vi "JSON Config Time Vector.vi"(7 "Expected Class":refnum<class "Abs_Time.lvclass">, 8 "error in (no error)":errorcluster, 11 "Test Value":timestamp) -> (0 "error out":errorcluster)   [LabVIEW 2021]
uses:
  Source/Abs_Types/Time/Abs_Time.lvclass
  C:/New folder/LV_Abstract/LV_Abstract/Source/Abs_Types/Type/Abs_Type.lvclass
  Source/Abs_Types/Time/Simple Read.vi
  Source/Constants/Support/Time/Time.vi
  <vilib>/addons/_JKI Toolkits/Caraya/classes/Assert/Assert Less_Variant.vi
  <vilib>/addons/_JKI Toolkits/Caraya/classes/Assert/Assert Equal Type_Variant.vi
  Source/Constants/Support/Time/Const_Time.lvclass
  <vilib>/addons/_JKI Toolkits/Caraya/classes/Assert/Assert.lvclass
  <vilib>/addons/_JKI Toolkits/Caraya/classes/Test/Test.lvclass
  <vilib>/Utility/Data Type/NI_Data Type.lvlib
  Source/Abs_Types/Type/Abs_Type.lvclass
panel:
  out "JSON":string
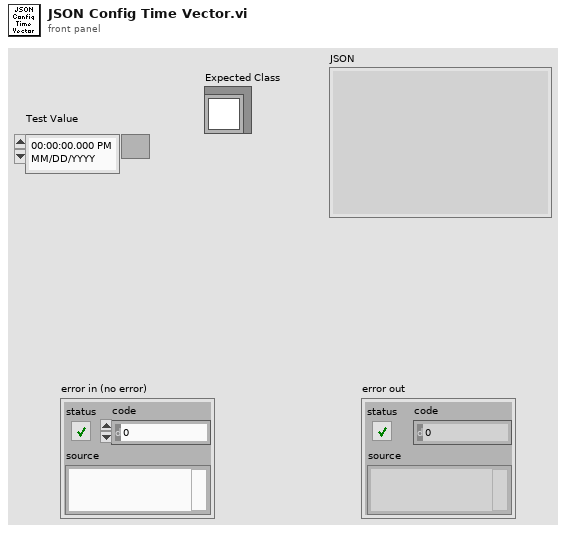
[diagram p1: front panel]
types:
  T1 = typedef "NI_Data Type.lvlib/Data Type.ctl" = enum8{"Invalid Type", "Void", "I8", "I16", "I32", "I64", "U8", "U16", "U32", "U64", "Single Float", "Double Float", "Extended Float", "Single Complex", "Double Complex", "Extended Complex", "Enum U8", "Enum U16", "Enum U32", "Enum U64", "Single Float With Unit", "Double Float With Unit", "Extended Float With Unit", "Single Complex with Unit", "Double Complex with Unit", "Extended Complex with Unit", "Boolean", "String", "Path", "Picture", "Tag", "Array", "Cluster", "Variant", "LV Variant", "Waveform", "Timestamp", "Digital Waveform", "Digital Data", "ExpressData", "Refnum", "External Data", "VI", "Poly VI", "LabVIEW Class Instance", "Fixed Point", "Set Collection", "Map Collection"}
  T2 = typedef "Abs_Time.lvclass/Type.ctl" = timestamp
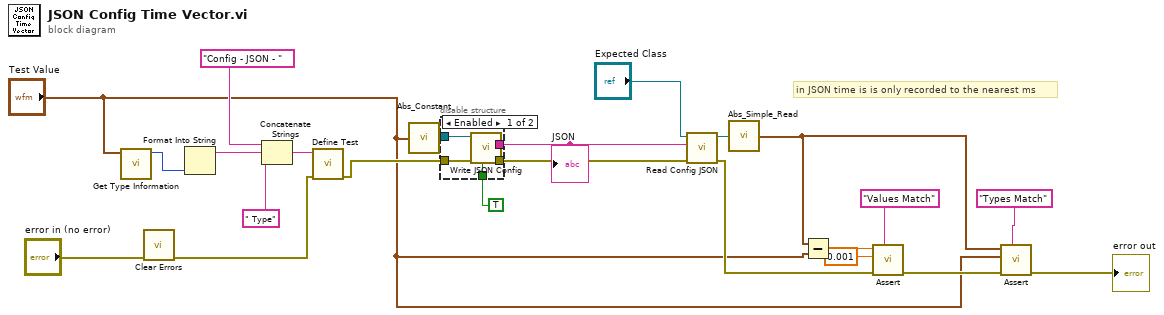
[diagram p0: block diagram]
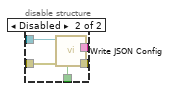
[diagram p2: hidden frame]
diagram:
  # "in JSON time is is only recorded to the nearest ms"
  n1 = call <vilib>:"Get Type Information.vi"("variant"="Test Value") -> ("type"=w14:T1)  [unwired: 6 in, 4 out]
  n2 = call <vilib>:"Clear Errors.vi"("error in (no error)"="error in (no error)") -> ("error out"=w9:errorcluster)  [unwired: 5 in, 1 out]
  n3 = Format Into String(w14) -> (resulting string=w13:string)  [unwired: 3 in, 1 out]
  n4 = Concatenate Strings("Config - JSON - " ("string"), w13, " Type" ("string")) -> (w12:string)
  n5 = call <vilib>:"Define Test.vi"("error in (no error)"=w9, "Label (VI Title)"=w12) -> ("error out"=w15:errorcluster)  [unwired: 8 in, 1 out]
  n6 = call-poly "Abs_Constant.vi"("Value"="Test Value") -> ("Constant"=w23:refnum<class "Const_Time.lvclass">)  [unwired: 4 in]
  n7 = disable-structure shown="Enabled" {
    disable-tunnel: w23 -> [w28 w33]
    disable-tunnel: TRUE ("Include Class Name") -> [w27 w32]
    disable-tunnel: [w26 w31] -> w21
    disable-tunnel: [w25 w30] -> w20
    disable-tunnel: w15 -> [w24 w29]
    frame Enabled {
      n8 = call-dynamic "Write JSON Config.vi"("Pretty Print?"=w27, "error in (no error)"=w24, "Const_Time in"=w28) -> ("error out"=w25:errorcluster, "JSON"=w26:string)  [unwired: 6 in, 1 out]
    }
    frame Disabled {
      n9 = call-dynamic "Write JSON Config.vi"("Pretty Print?"=w32, "error in (no error)"=w29, "Const_Time in"=w33) -> ("error out"=w30:errorcluster, "JSON"=w31:string)  [unwired: 6 in, 1 out]
    }
  }
  "JSON" <- w21
  n10 = call "Read Config JSON.vi"("error in (no error)"=w20, "JSON Config"=w21, "Abs_Type in"="Expected Class") -> ("error out"=w18:errorcluster, "Abs_Type out"=w19:refnum<class "Abs_Time.lvclass">)  [unwired: 7 in]
  n11 = call-poly "Abs_Simple_Read.vi"("Class"=w19) -> ("Value"=w3:T2)  [unwired: 4 in]
  n12 = Subtract(x=w3, y="Test Value") -> (x-y=w2:dbl)
  n13 = call-poly <vilib>:"Assert.vi"("Label"="Values Match", "error in (no error)"=w18, "Actual"=0.001, "Expected"=w2) -> ("error out"=w7:errorcluster)  [unwired: 6 in, 1 out]
  n14 = call-poly <vilib>:"Assert.vi"("Label"="Types Match", "error in (no error)"=w7, "Actual"="Test Value", "Expected"=w3) -> ("error out"=→"error out":errorcluster)  [unwired: 6 in, 1 out]
